vi "AddListenerMailbox.vi"(8 "error in (no error)":errorcluster, 10 "Message Enqueuer":refnum<class "Message Enqueuer.lvclass">, 11 "MailboxManager in":refnum<class "MailboxManager.lvclass">) -> (0 "error out":errorcluster, 3 "MailboxManager out":refnum<class "MailboxManager.lvclass">)   [LabVIEW 2020, in "MailboxManager.lvlib" / "MailboxManager.lvclass"]
uses:
  MailboxManager.lvclass
  MailBoxMessage/MailBoxMessage.lvclass
  <vilib>/ActorFramework/Message Enqueuer/Message Enqueuer.lvclass
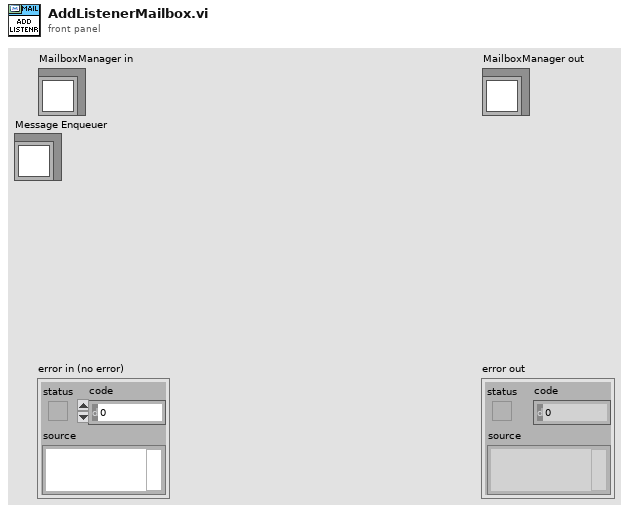
[diagram p1: front panel]
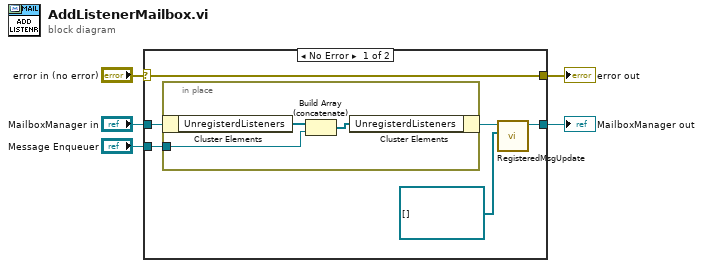
[diagram p0: block diagram]
diagram:
  n1 = case shown="No Error" "error in (no error)" {
    selector: "error in (no error)" -> [w11 w16]
    tunnel: [w11 w16] -> w4
    tunnel: [w7 w15] -> w2
    tunnel: "MailboxManager in" -> [w10 w15]
    tunnel: "Message Enqueuer" -> [w9 _]
    frame No Error {
      n2 = in-place {
        in-place-border: w9 -> [w12]
        n3 = in-place-cluster #1(w10) -> ("UnregisterdListeners"=w14:refnum<class "Message Enqueuer.lvclass">[])
        n4 = Build Array (concatenate)(w14, w12) -> (w13:refnum<class "Message Enqueuer.lvclass">[])
        n5 = in-place-cluster #1("UnregisterdListeners"=w13) -> (w8:refnum<class "MailboxManager.lvclass">)
      }
      n6 = call-dynamic "RegisteredMsgUpdate.vi"("Msgs"=refnum<class "MailBoxMessage.lvclass">[] [], "MailboxManager in"=w8) -> ("MailboxManager out"=w7:refnum<class "MailboxManager.lvclass">)  [unwired: 8 in, 1 out]
    }
    frame Error {
    }
  }
  "error out" <- w4
  "MailboxManager out" <- w2
